vi "RSNRPZpid.vi"(7 "RSNPRZsettings":refnum<vi>, 11 "av power in":dbl format="%#_13g") -> ()   [LabVIEW 2019]
uses:
  RSNRPZcontrol.ctl
  <vilib>/Utility/error.llb/Error Cluster From Error Code.vi
  <vilib>/rvi/errors/niLvFpgaAdjustHostInterfaceError.vi
  <vilib>/addons/control/pid/pid.llb/PID (DBL).vi
  <vilib>/rvi/interface/nirviReadWriteControl/nirviReadWriteControl.xnode
  <vilib>/addons/control/pid/NI_PID_pid.lvlib
  NiFpgaLv.dll
  <vilib>/rvi/interface/Simulation/niFpgaSimulationCallBeginRW.vi
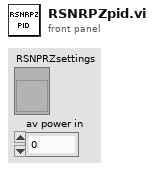
[diagram p1: front panel]
types:
  T1 = typedef "RSNRPZcontrol.ctl" = cluster{"Average Counts :":dbl, "Correction Freq [MHz] :":dbl, "Integration Time [ms] : ":dbl, "P :":dbl, "I :":dbl, "D :":dbl, "Power setpoint :":dbl, "PID on :":bool, "Voltage :":dbl, "Reset :":bool, "Agilient Power Level [dBm] :":dbl}
  T2 = cluster{"proportional gain (Kc)":dbl, "integral time (Ti, min)":dbl, "derivative time (Td, min)":dbl}
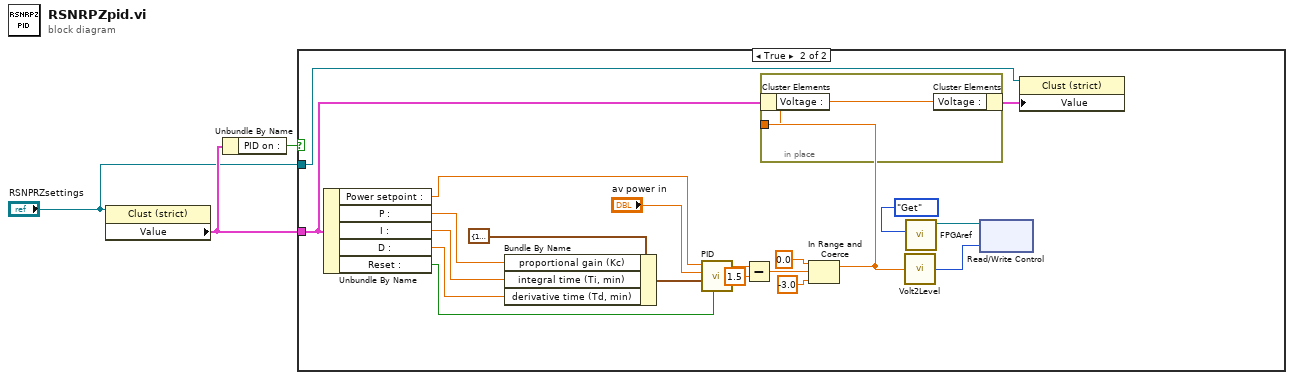
[diagram p0: block diagram]
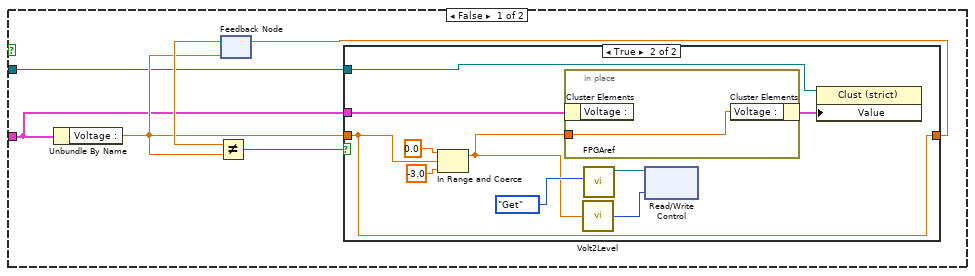
[diagram p2: hidden frame]
diagram:
  n1 = property class="Clust (strict)"(reference="RSNPRZsettings") -> ("Value"=w2:T1)  [unwired: 1 in, 2 out]
  n2 = Unbundle By Name(w2) -> ("PID on :"=w3:bool)
  n3 = case shown="True" w3 {
    tunnel: w2 -> [w5 w32]
    tunnel: "RSNPRZsettings" -> [w4 w30]
    frame False {
      n4 = Unbundle By Name(w5) -> ("Voltage :"=w7:dbl)
      n5 = feedback #1(w7) -> (w9:dbl)
      n6 = Not Equal?(x=w9, y=w7) -> (x != y?=w8:bool)
      n7 = case shown="True" w8 {
        tunnel: w7 -> [w10 w17]
        tunnel: [w10 w17] -> w6
        tunnel: w5 -> [_ w14]
        tunnel: w4 -> [_ w12]
        frame False {
        }
        frame True {
          n8 = In Range and Coerce(upper limit=0.0, x=w17, lower limit=-3.0) -> (coerced(x)=w13:dbl)  [unwired: 1 out]
          n9 = in-place {
            in-place-border: w13 -> [w21]
            n10 = in-place-cluster #2(w14) -> ()  [unwired: 1 out]
            n11 = in-place-cluster #2("Voltage :"=w21) -> (w11:T1)
          }
          n12 = call "Volt2Level.vi"("voltage /V"=w13) -> ("level"=w18:i16)
          n13 = call "FPGAref.vi"("Enum"=enum16{"Set", "Get"}."Get") -> ("FPGA VI Reference Out 2"=w19:refnum<k20>)  [unwired: 5 in, 1 out]
          n14 = xnode "Read/Write Control"("FPGA VI Reference In"=w19, "AO5"=w18) -> ()  [unwired: 1 in, 2 out]
          n15 = property class="Clust (strict)"(reference=w12, "Value"=w11) -> ()  [unwired: 1 in, 2 out]
        }
      }
      n16 = feedback-in #1(w6) -> ()
    }
    frame True {
      n17 = Unbundle By Name(w32) -> ("Power setpoint :"=w36:dbl, "P :"=w39:dbl, "I :"=w38:dbl, "D :"=w37:dbl, "Reset :"=w28:bool)
      n18 = Bundle By Name(cluster=T2 {"proportional gain (Kc)"=1.0, "integral time (Ti, min)"=0.01, "derivative time (Td, min)"=0.0} ("PID gains"), "proportional gain (Kc)"=w39, "integral time (Ti, min)"=w38, "derivative time (Td, min)"=w37) -> (w40:T2)
      n19 = call-poly <vilib>:"PID.vi"("reinitialize? (F)"=w28, "PID gains"=w40, "process variable"="av power in", "setpoint"=w36) -> ("output"=w27:dbl)  [unwired: 6 in, 1 out]
      n20 = Subtract(x=w27, y=1.5) -> (x-y=w23:dbl)
      n21 = In Range and Coerce(upper limit=0.0, x=w23, lower limit=-3.0) -> (coerced(x)=w22:dbl)  [unwired: 1 out]
      n22 = in-place {
        in-place-border: w22 -> [w42]
        n23 = in-place-cluster #3(w32) -> ()  [unwired: 1 out]
        n24 = in-place-cluster #3("Voltage :"=w42) -> (w29:T1)
      }
      n25 = call "Volt2Level.vi"("voltage /V"=w22) -> ("level"=w31:i16)
      n26 = call "FPGAref.vi"("Enum"=enum16{"Set", "Get"}."Get") -> ("FPGA VI Reference Out 2"=w33:refnum<k20>)  [unwired: 5 in, 1 out]
      n27 = xnode "Read/Write Control"("FPGA VI Reference In"=w33, "AO5"=w31) -> ()  [unwired: 1 in, 2 out]
      n28 = property class="Clust (strict)"(reference=w30, "Value"=w29) -> ()  [unwired: 1 in, 2 out]
    }
  }
